vi "Main.vi"() -> ()   [LabVIEW 2011]
uses:
  typedefs/fiber_parameters_cluster.ctl
  fpga/typedefs/ramp_type_enum.ctl
  typedefs/spiral_parameters_cluster.ctl
  typedefs/run_parameters_cluster.ctl
  typedefs/run_mode_enum.ctl
  typedefs/acquisition_parameters_cluster.ctl
  typedefs/image_size_I32.ctl
  typedefs/scan_infos.ctl
  typedefs/smooth_coeffs_cluster.ctl
  typedefs/storage_parameters_cluster.ctl
  typedefs/mapping_corrections_cluster.ctl
  typedefs/pockels_corrections_cluster.ctl
  typedefs/fiber_parameters_pixelmapper_autoupdate_cluster.ctl
  typedefs/main_state_cluster.ctl
  typedefs/main_state_enum.ctl
  typedefs/control_process_state_cluster.ctl
  typedefs/control_process_state_enum.ctl
  typedefs/state_insert_position_enum.ctl
  <vilib>/Utility/error.llb/DialogType.ctl
  typedefs/all_scan_parameters_cluster.ctl
  <vilib>/DAQmx/write.llb/DAQmx Write (Digital Bool 1Line 1Point).vi
  globals/global_process_names.vi
  globals/global_exit.vi
  <vilib>/DAQmx/create/channels.llb/DAQmx Create Channel (DO-Digital Output).vi
  <vilib>/DAQmx/miscellaneous.llb/DAQmx Fill In Error Info.vi
  Fiberscope_library.lvlib
panel:
  out "Loaded process names":string[](array[string])
  in  "PMT":bool
  out "Version_string":string
  out "Loading":i32(slide) scale=0.0..6.0
  out "CPU":sgl(slide) scale=0.0..100.0
  in  "Comment":string
  in  "Save":bool
  in  "Start single":bool
  in  "Shutter":bool
  in  "Parameters":T1(tab)
  in  "Fiber parameters":T2={"Frequency"=2039.0, "Amplitude X"=0.3, "Amplitude Y"=0.3, "Initial Amplitude X"=0.0, "Initial Amplitude Y"=0.0, "Phase"=0.0, "Ramp type"=enum."Linear"} {"Phase" min=-90.0 max=90.0 step=5.0; "Initial Amplitude Y" min=0.0 max=1.0 step=0.1; "Initial Amplitude X" min=0.0 max=1.0 step=0.1; "Amplitude Y" min=0.0 max=4.0 step=0.1; "Amplitude X" min=0.0 max=4.0 step=0.1; "Frequency" min=100.0 max=6000.0 step=1.0}
  in  "Spiral parameters":T4={"Imaging periods"=100.0, "Settling periods"=50.0, "Resting periods"=100.0} {"Resting periods" min=10.0 max=1000.0 step=1.0; "Settling periods" min=1.0 max=1000.0 step=1.0; "Imaging periods" min=1.0 max=1000.0 step=1.0}
  in  "Run parameters":T5={"Run mode"=enum."Continuous", "Averages per frame"=1, "No. of frames"=1} {"No. of frames" min=1 max=1000 step=1; "Averages per frame" min=1 max=32}
  in  "Acquisition parameters":T7={"Cycles per pixel"=391, "Image size"=128, "Bidirectional acquisition"=FALSE} {"Image size" items=["128x128 px"=128, "256x256 px"=256, "512x512 px"=512]; "Cycles per pixel" min=100 max=90000 step=1}
  out "Scan infos":T9 {"Scan vs. Non-scan" scale=0.0..1.0}
  in  "Pockels corrections":T10 {"Delay pixels" min=0 max=10000 step=1}
  in  "Smoothing coefficients":T11 {"Coeff 1" min=0.0 max=1.0 step=0.05; "Coeff 2" min=0.0 max=1.0 step=0.05}
  in  "Fiber parameters pixelmapper":T2={"Frequency"=2039.0, "Amplitude X"=0.3, "Amplitude Y"=0.3, "Initial Amplitude X"=0.0, "Initial Amplitude Y"=0.0, "Phase"=0.0, "Ramp type"=enum."Linear"} {"Phase" min=-90.0 max=90.0 step=5.0; "Initial Amplitude Y" min=0.0 max=1.0 step=0.1; "Initial Amplitude X" min=0.0 max=1.0 step=0.1; "Amplitude Y" min=0.0 max=4.0 step=0.1; "Amplitude X" min=0.0 max=4.0 step=0.1; "Frequency" min=100.0 max=6000.0 step=1.0}
  in  "Mapping corrections":T12 {"Phase increase" min=-1.0 max=1.0 step=0.01}
  in  "Autoupdate":T13
  in  "Storage parameters":T14
  in  "PMT digital line":tag="PXI-6229/port0/line1"
  in  "Shutter digital line":tag="PXI-6229/port0/line0"
  in  "Start cont":bool
  in  "Quit":bool
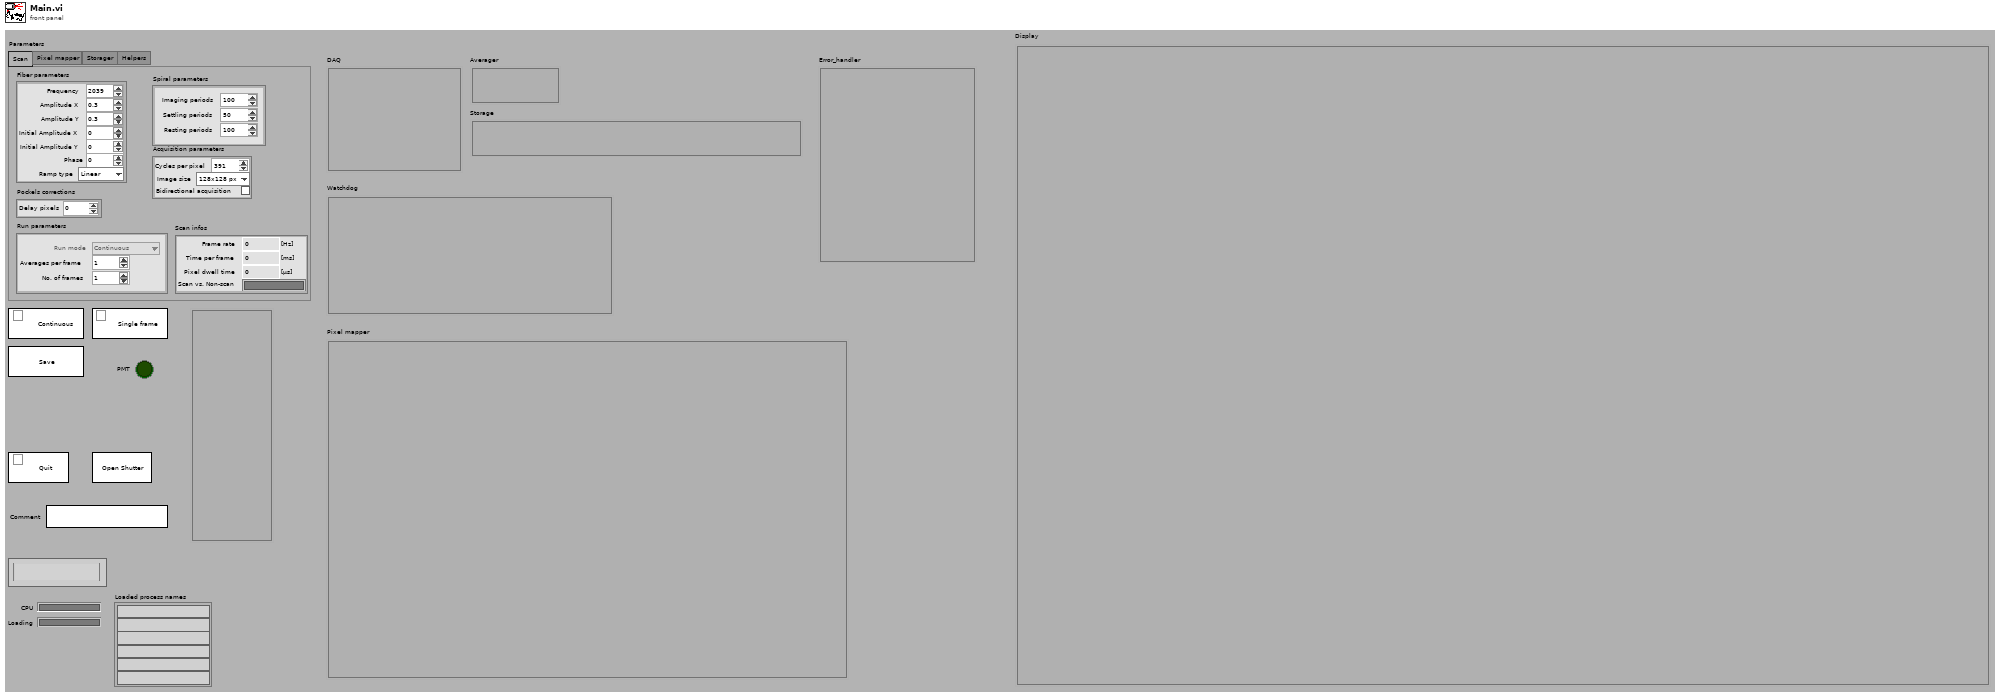
[diagram p1: front panel]
types:
  T1 = enum32{"Scan", "Pixel mapper", "Storager", "Helpers"}
  T2 = typedef "Fiberscope_library.lvlib/fiber_parameters_cluster.ctl" = cluster{"Frequency":dbl, "Amplitude X":dbl, "Amplitude Y":dbl, "Initial Amplitude X":dbl, "Initial Amplitude Y":dbl, "Phase":dbl, "Ramp type":T3}
  T3 = typedef "ramp_type_enum.ctl" = enum8{"Linear", "Sine"}
  T4 = typedef "Fiberscope_library.lvlib/spiral_parameters_cluster.ctl" = cluster{"Imaging periods":dbl, "Settling periods":dbl, "Resting periods":dbl}
  T5 = typedef "Fiberscope_library.lvlib/run_parameters_cluster.ctl" = cluster{"Run mode":T6, "Averages per frame":u8, "No. of frames":u32}
  T6 = typedef "Fiberscope_library.lvlib/run_mode_enum.ctl" = enum16{"Continuous", "Single frame", "No. of frames"}
  T7 = typedef "Fiberscope_library.lvlib/acquisition_parameters_cluster.ctl" = cluster{"Cycles per pixel":u32, "Image size":T8, "Bidirectional acquisition":bool}
  T8 = typedef "Fiberscope_library.lvlib/image_size_I32.ctl" = i32
  T9 = typedef "Fiberscope_library.lvlib/scan_infos.ctl" = cluster{"Frame rate":dbl, "Pixel dwell time":dbl, "Scan vs. Non-scan":dbl, "Time per frame":dbl}
  T10 = typedef "Fiberscope_library.lvlib/pockels_corrections_cluster.ctl" = cluster{"Delay pixels":i32}
  T11 = typedef "Fiberscope_library.lvlib/smooth_coeffs_cluster.ctl" = cluster{"Coeff 1":dbl, "Coeff 2":dbl}
  T12 = typedef "Fiberscope_library.lvlib/mapping_corrections_cluster.ctl" = cluster{"Phase increase":dbl, "Amplitude correction":dbl}
  T13 = typedef "Fiberscope_library.lvlib/fiber_parameters_pixelmapper_autoupdate_cluster.ctl" = cluster{"Frequency":bool, "Amplitude X":bool, "Amplitude Y":bool, "Initial Amplitude X":bool, "Initial Amplitude Y":bool, "Phase":bool, "Ramp type":bool}
  T14 = typedef "Fiberscope_library.lvlib/storage_parameters_cluster.ctl" = cluster{"Autosave":bool, "Path":path}
  T15 = typedef "Fiberscope_library.lvlib/main_state_cluster.ctl" = cluster{"Main_state_enum":T16, "State_data_variant":variant}
  T16 = typedef "Fiberscope_library.lvlib/main_state_enum.ctl" = enum16{"Init", "Error", "Quit", "Run", "Stop", "Change_parameters", "Timeout", "Shutter", "Save", "Wait_for_finished", "Change_storage", "Change_pixelmap", "Change_averages", "Run_finished", "Change_runmode", "PMT"}
  T17 = cluster{"Quit":refnum<vi>, "Start cont":refnum<vi>, "Parameters":refnum<vi>, "Fiber parameters":refnum<vi>, "Spiral parameters":refnum<vi>, "Run parameters":refnum<vi>, "Acquisition parameters":refnum<vi>, "Fiber parameters pixelmapper":refnum<vi>, "Shutter":refnum<vi>, "Save":refnum<vi>, "Comment":refnum<vi>, "Start single":refnum<vi>, "Storage parameters":refnum<vi>, "PMT":refnum<vi>}
  T18 = typedef "Fiberscope_library.lvlib/all_scan_parameters_cluster.ctl" = cluster{"Fiber parameters":T2, "Spiral parameters":T4, "Run parameters":T5, "Acquisition parameters":T7, "Fiber parameters pixel_mapper":T2, "Smooth_coeffs_cluster":T11, "Storage parameters":T14, "Mapping corrections":T12, "Pockels corrections":T10}
  T19 = cluster{"Mapping corrections":T12, "Smoothing coefficients":T11, "Fiber parameters pixelmapper":T2}
  T20 = typedef "Fiberscope_library.lvlib/control_process_state_cluster.ctl" = cluster{"Control_process_state_enum":T21, "variant":variant}
  T21 = typedef "Fiberscope_library.lvlib/control_process_state_enum.ctl" = enum16{"Init", "Quit", "Start", "Stop", "Change_parameters", "Running", "Finish", "Custom"}
  T22 = typedef "Fiberscope_library.lvlib/state_insert_position_enum.ctl" = enum16{"Insert_back", "Insert_front"}
  T23 = cluster{"error in (no error)":errorcluster, string}
  T24 = enum8{"Enabled", "Disabled", "Disabled and Grayed Out"}
  T25 = typedef "DialogType.ctl" = u16
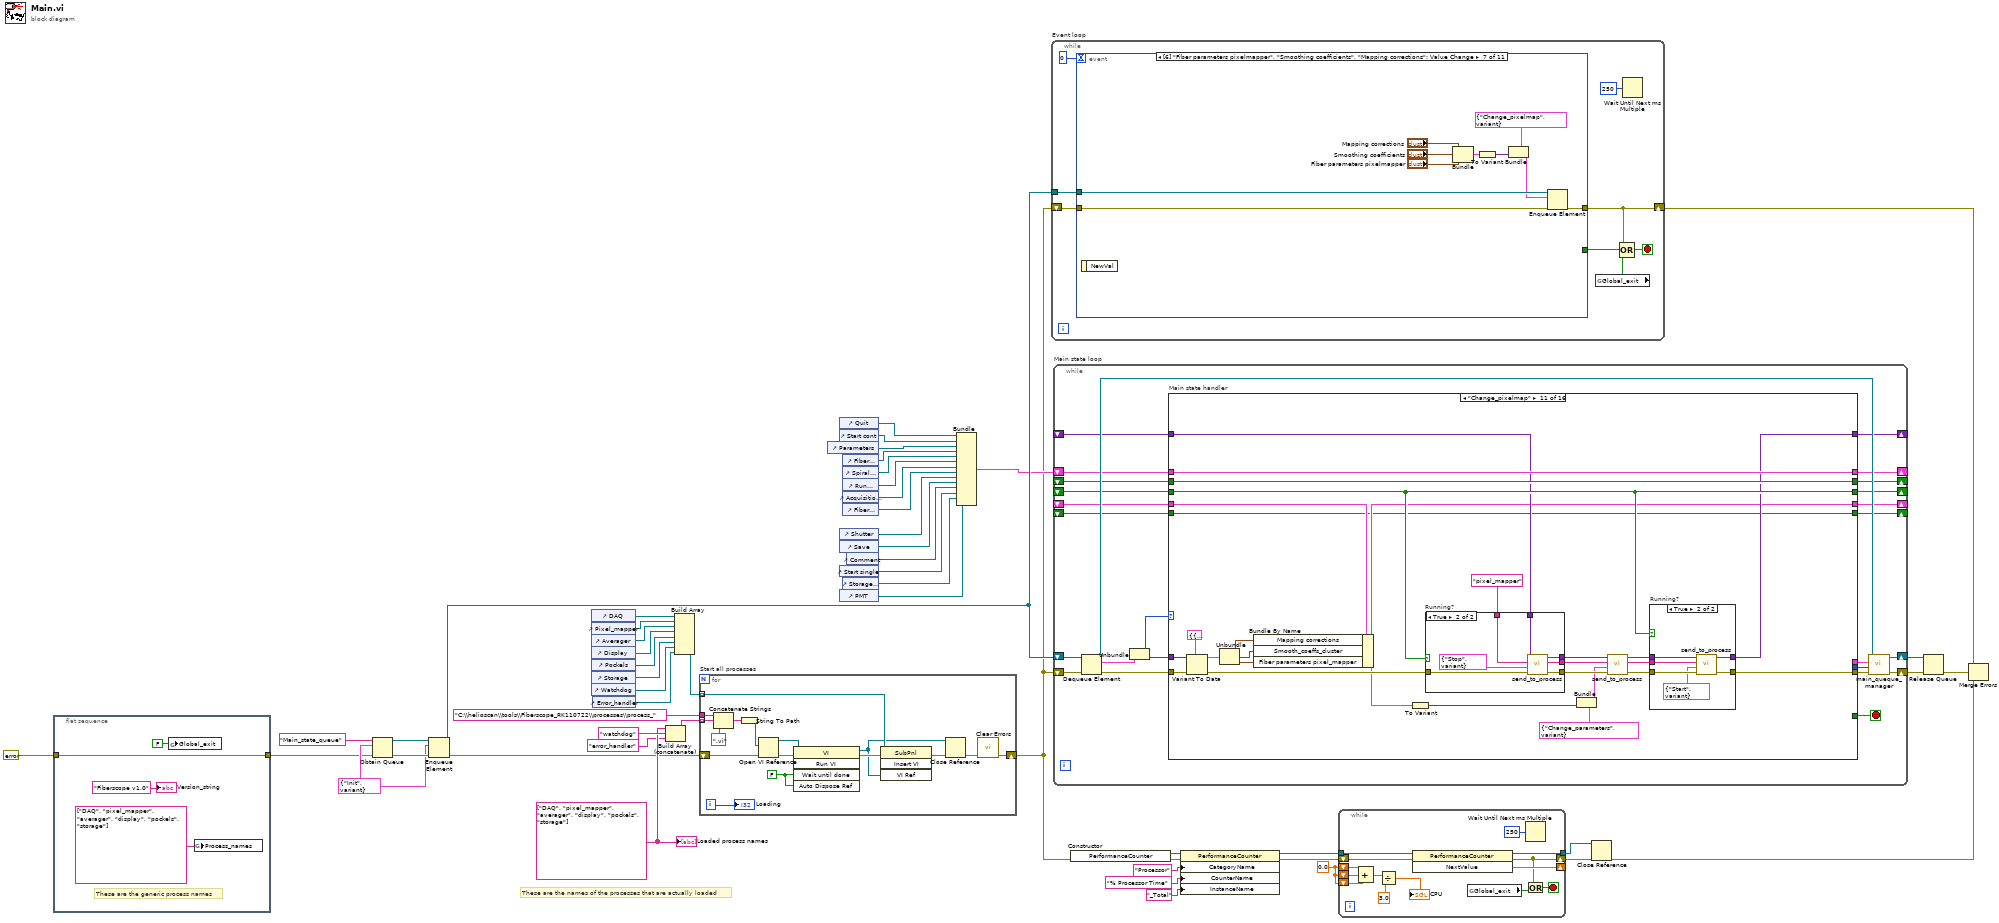
[diagram p0: block diagram]
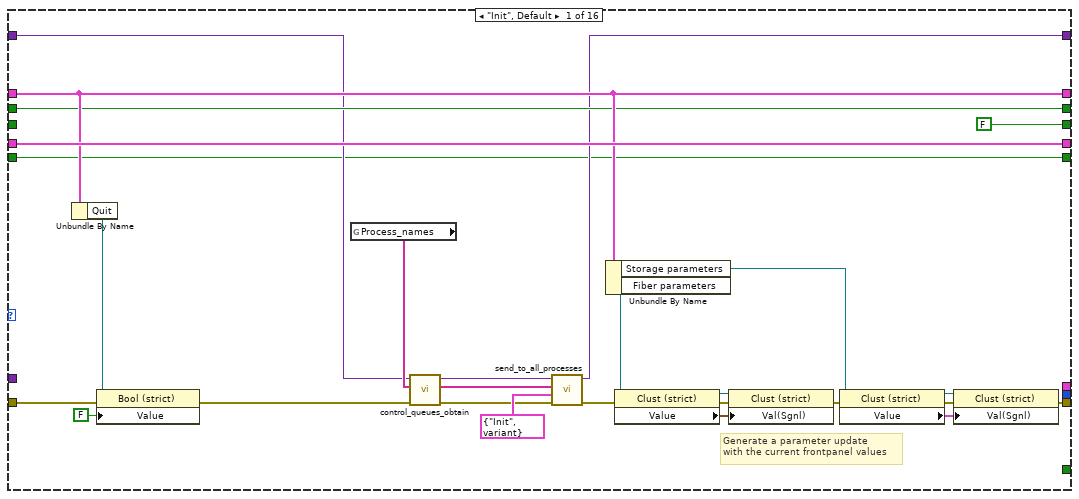
[diagram p2: hidden frame]
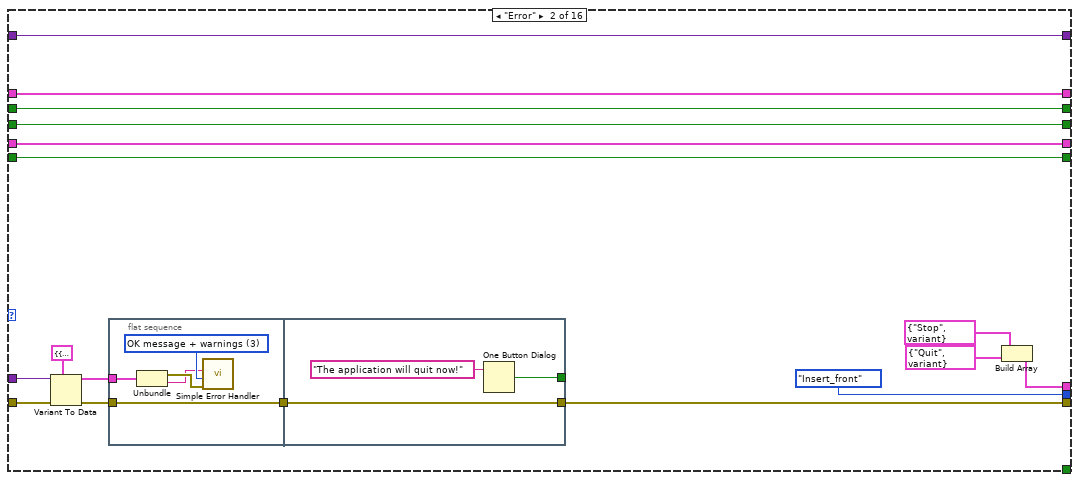
[diagram p3: hidden frame]
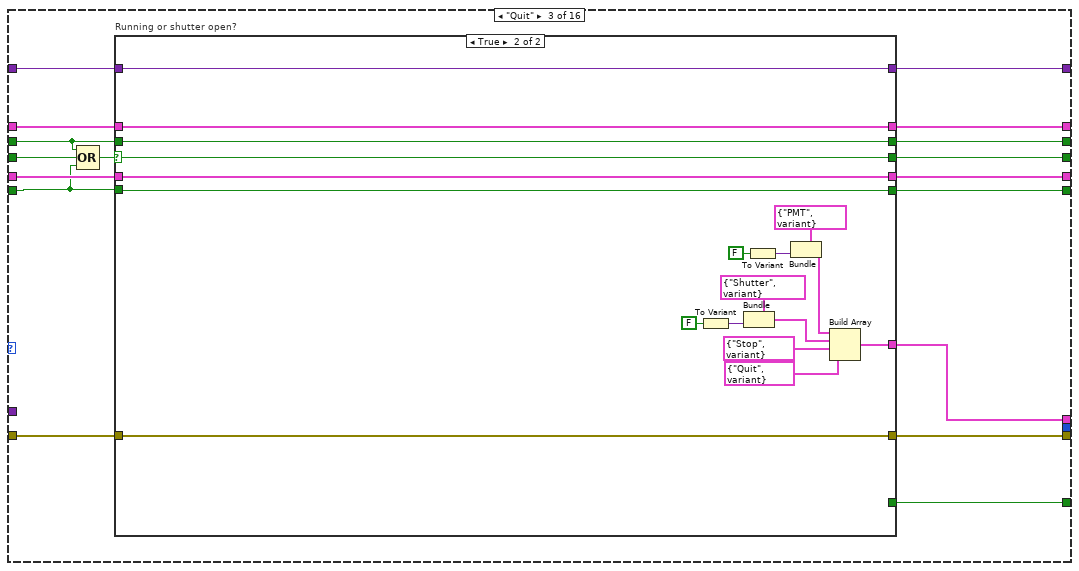
[diagram p4: hidden frame]
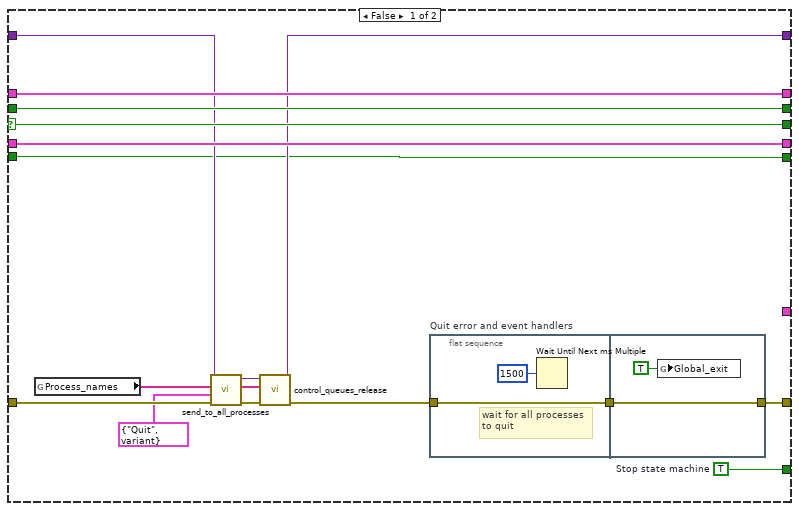
[diagram p5: hidden frame]
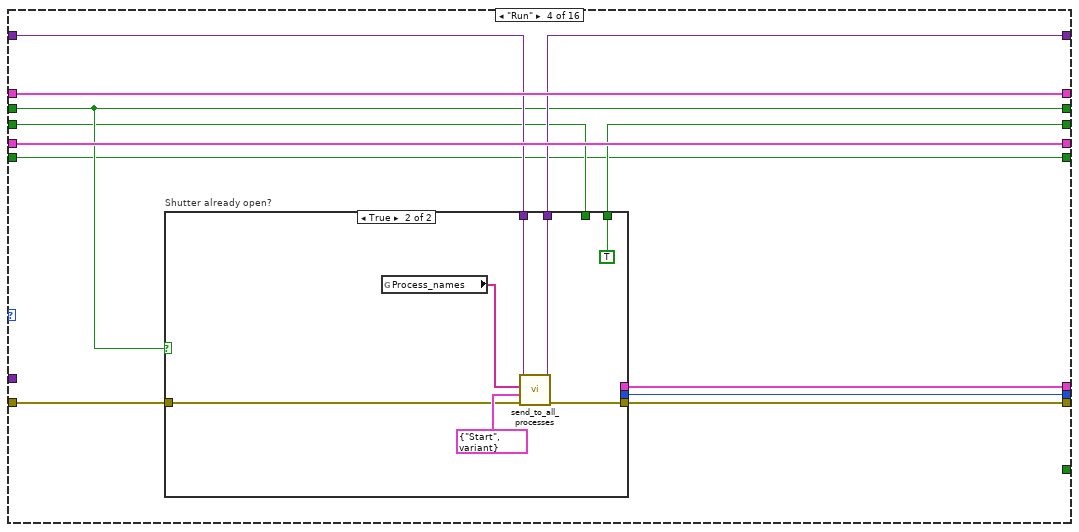
[diagram p6: hidden frame]
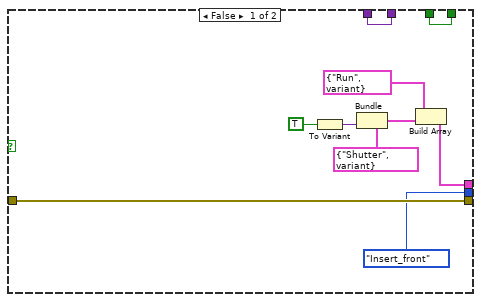
[diagram p7: hidden frame]
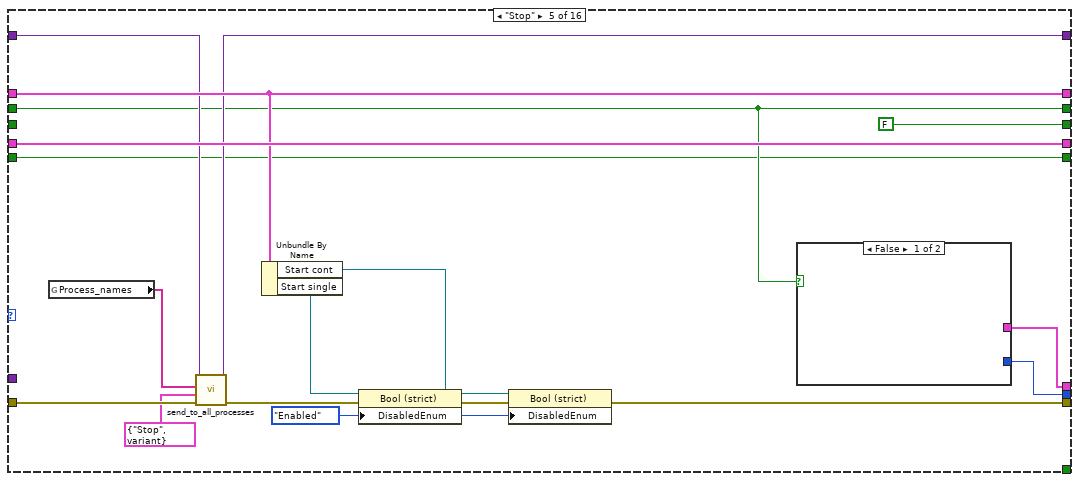
[diagram p8: hidden frame]
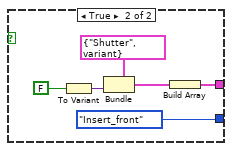
[diagram p9: hidden frame]
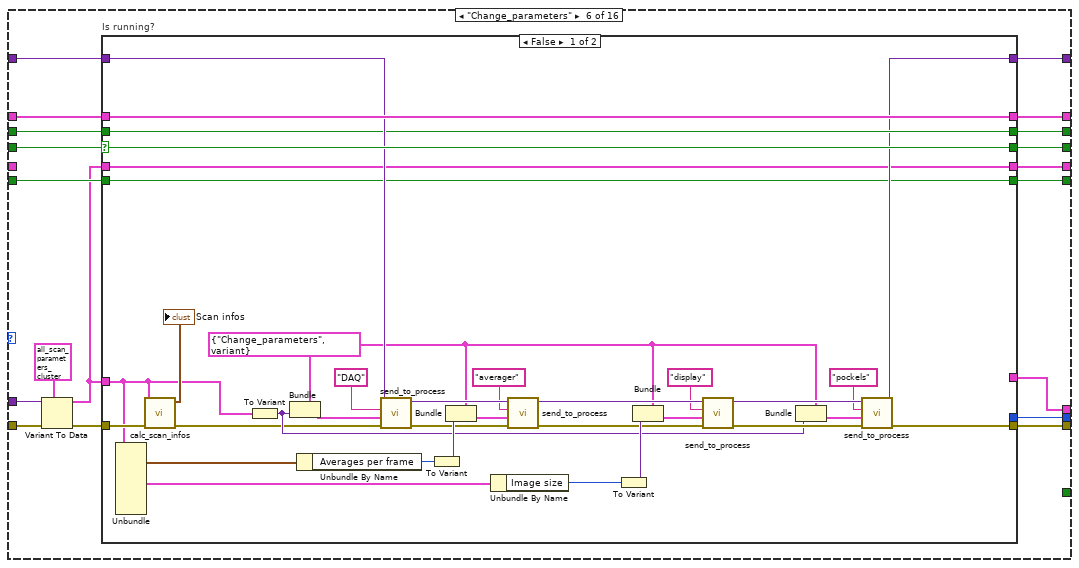
[diagram p10: hidden frame]
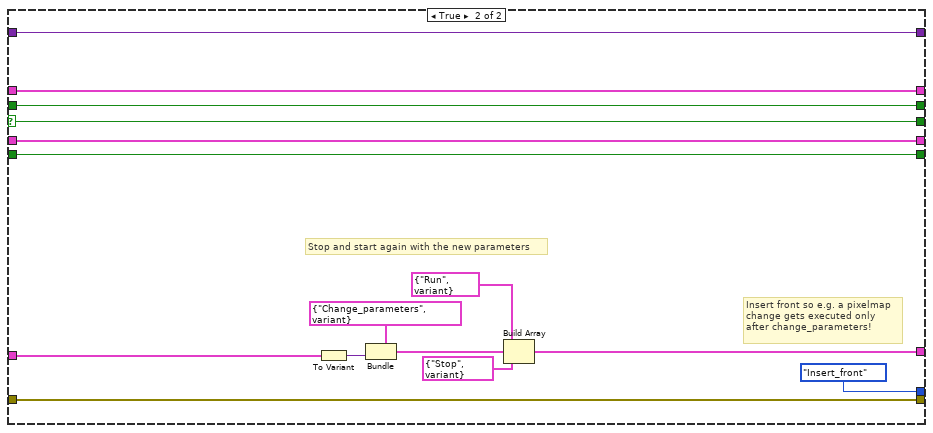
[diagram p11: hidden frame]
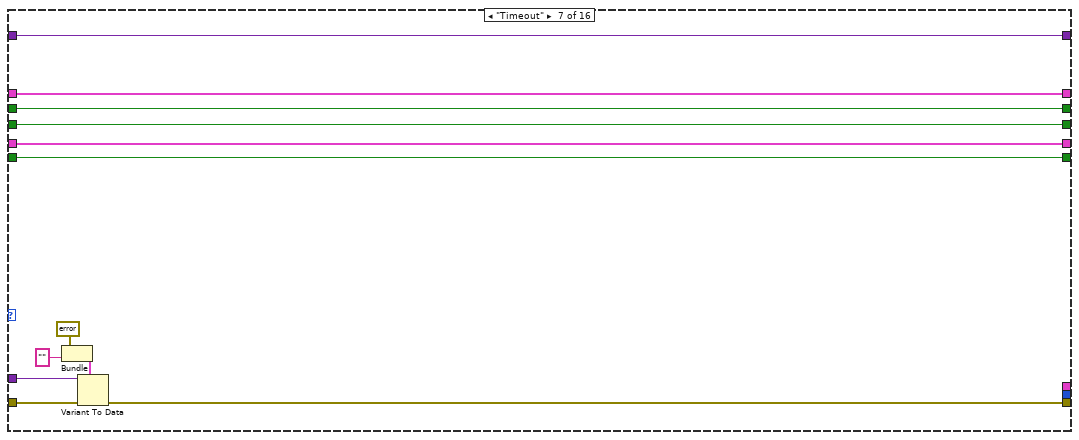
[diagram p12: hidden frame]
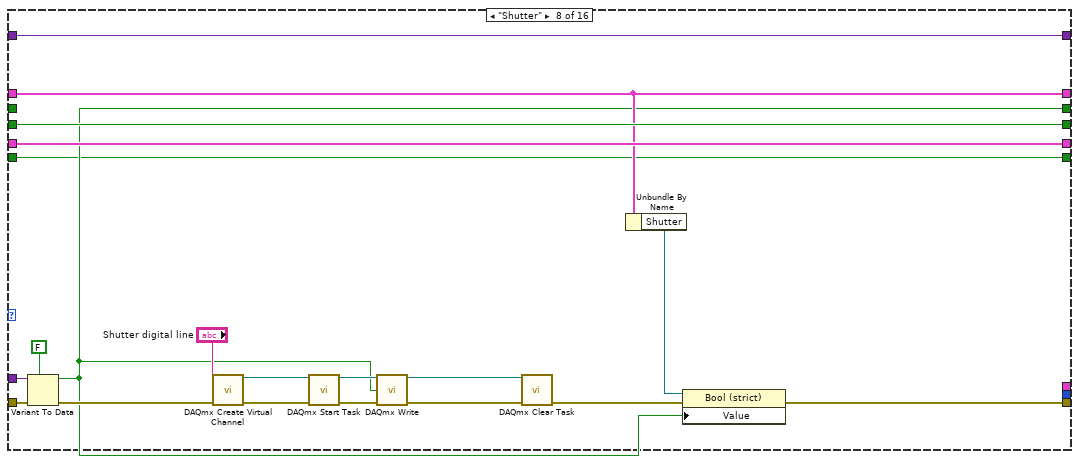
[diagram p13: hidden frame]
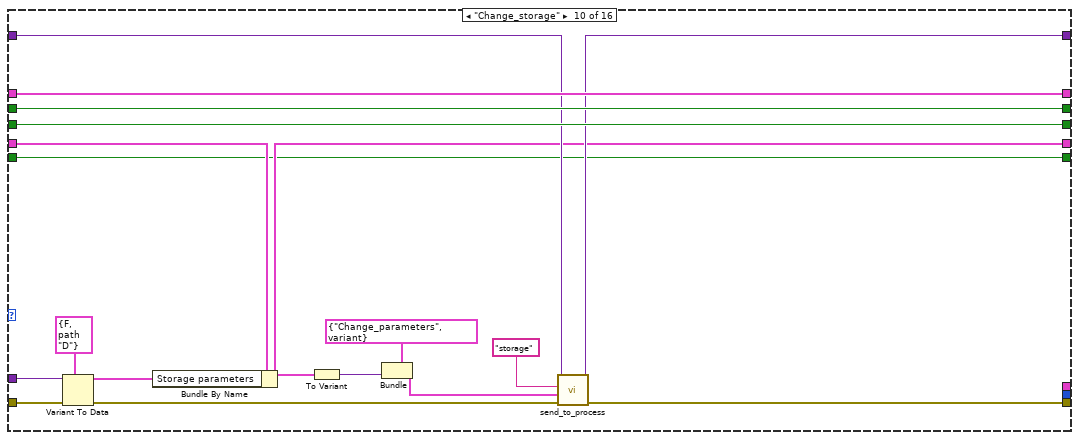
[diagram p15: hidden frame]
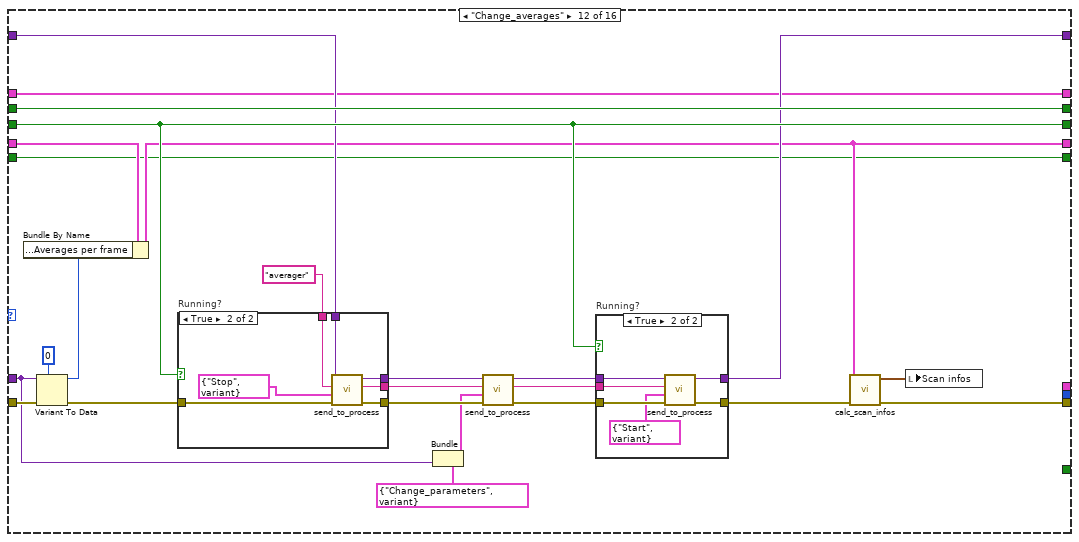
[diagram p18: hidden frame]
diagram:
  w10 = string[] ["DAQ", "pixel_mapper", "averager", "display", "pockels", "storage"]
  w22 = sgl 0.0 ("NextValue")
  w49 = T15 {"Main_state_enum"=enum."Init", "State_data_variant"=variant} ("Main_state_cluster")
  # "These are the names of the processes that are actually loaded"
  n1 = flat-sequence {
    tunnel: [w56] -> w37
    tunnel: errorcluster {"status"=FALSE, "code"=0, "source"=""} ("error in (no error)") -> [w56]
    frame #0 {
      # "These are the generic process names"
      n2 = global write "global_exit.vi" "Global_exit"(FALSE ("Global_exit")) -> ()
      n3 = global write "global_process_names.vi" "Process_names"(string[] ["DAQ", "pixel_mapper", "averager", "display", "pockels", "storage"]) -> ()
      "Version_string" <- "Fiberscope v1.0" ("Version_string")
    }
  }
  n4 = Obtain Queue(name (unnamed)="Main_state_queue", element data type=w49, error in (no error)=w37) -> (queue out=w51:refnum<queue>, error out=w52:errorcluster)  [unwired: 2 in, 1 out]
  n5 = Enqueue Element(queue=w51, element=w49, error in (no error)=w52) -> (queue out=w50:refnum<queue>, error out=w8:errorcluster)  [unwired: 1 in, 1 out]
  n6 = control-ref of="DAQ"() -> (w19:refnum<vi>)
  n7 = control-ref of="Pixel_mapper"() -> (w18:refnum<vi>)
  n8 = control-ref of="Averager"() -> (w17:refnum<vi>)
  n9 = control-ref of="Display"() -> (w16:refnum<vi>)
  n10 = control-ref of="Pockels"() -> (w14:refnum<vi>)
  n11 = control-ref of="Storage"() -> (w13:refnum<vi>)
  n12 = control-ref of="Watchdog"() -> (w12:refnum<vi>)
  n13 = control-ref of="Error_handler"() -> (w4:refnum<vi>)
  n14 = Build Array (concatenate)(w10, "watchdog", "error_handler" ("element")) -> (w9:string[])
  n15 = Build Array(w19, w18, w17, w16, w14, w13, w12, w4) -> (w15:refnum<vi>[])
  n16 = for "Start all processes" {
    tunnel: w9 -> [w71] mode=indexing
    tunnel: w15 -> [w73] mode=indexing
    tunnel: "C:\\helioscan\\tools\\Fiberscope_RK110722\\processes\\process_" -> [w72]
    shift-right: [w66] -> w6
    shift-left: w8 -> [w67]
    i -> [w58]
    w59 = FALSE
    n17 = Concatenate Strings(w72, w71, ".vi") -> (w69:string)
    n18 = String To Path(string=w69) -> (path=w68:path)
    n19 = Open VI Reference(vi path=w68, error in (no error)=w67) -> (vi reference=w61:refnum<vi>, error out=w63:errorcluster)  [unwired: 4 in]
    n20 = invoke class="VI" method="Run VI"(reference=w61, error in=w63, "Wait until done"=w59, "Auto Dispose Ref"=w59) -> (reference out=w60:refnum<vi>, error out=w62:errorcluster)  [unwired: 1 in, 3 out]
    n21 = invoke class="SubPnl" method="Insert VI"(reference=w73, error in=w62, "VI Ref"=w60) -> (error out=w65:errorcluster)  [unwired: 1 in, 3 out]
    n22 = Close Reference(reference=w60, error in (no error)=w65) -> (error out=w64:errorcluster)
    n23 = call <vilib>:"Clear Errors.vi"("error in (no error)"=w64) -> ("error out"=w66:errorcluster)  [unwired: 6 in]
    "Loading" <- w58
  }
  n24 = control-ref of="Parameters"() -> (w46:refnum<vi>)
  n25 = control-ref of="Quit"() -> (w48:refnum<vi>)
  n26 = control-ref of="Start cont"() -> (w47:refnum<vi>)
  n27 = control-ref of="Shutter"() -> (w34:refnum<vi>)
  n28 = control-ref of="Save"() -> (w33:refnum<vi>)
  n29 = control-ref of="Start single"() -> (w30:refnum<vi>)
  n30 = control-ref of="PMT"() -> (w1:refnum<vi>)
  n31 = control-ref of="Fiber parameters"() -> (w45:refnum<vi>)
  n32 = control-ref of="Spiral parameters"() -> (w44:refnum<vi>)
  n33 = control-ref of="Run parameters"() -> (w43:refnum<vi>)
  n34 = control-ref of="Acquisition parameters"() -> (w31:refnum<vi>)
  n35 = control-ref of="Fiber parameters pixelmapper"() -> (w35:refnum<vi>)
  n36 = control-ref of="Storage parameters"() -> (w3:refnum<vi>)
  n37 = control-ref of="Comment"() -> (w32:refnum<vi>)
  n38 = Bundle("Quit"=w48, "Start cont"=w47, "Parameters"=w46, "Fiber parameters"=w45, "Spiral parameters"=w44, "Run parameters"=w43, "Acquisition parameters"=w31, "Fiber parameters pixelmapper"=w35, "Shutter"=w34, "Save"=w33, "Comment"=w32, "Start single"=w30, "Storage parameters"=w3, "PMT"=w1) -> (w42:T17)  [unwired: 1 in]
  n39 = while "Event loop" {
    tunnel: w50 -> [w81]
    shift-right: [w74] -> w38
    shift-left: w6 -> [w80]
    stop <- w79 stop-if-true
    n40 = event shown="[6] \"Fiber parameters pixelmapper\", \"Smoothing coefficients\", \"Mapping corrections\": Value Change" {
      selector: _ -> [_ _ _ _ _ _ _ _ _ _ _]
      dyn-events: _ -> [_ _ _ _ _ _ _ _ _ _ _]
      timeout: 0 -> [_ _ _ _ _ _ _ _ _ _ _]
      tunnel: w81 -> [_ w84 w89 w113 w140 w145 w158 w161 w176 _ w184]
      tunnel: w80 -> [w82 w86 w90 w115 w125 w149 w150 w163 w178 w179 w186]
      tunnel: [w82 w85 w88 w114 w130 w146 w159 w162 w177 w179 w185] -> w74
      tunnel: [_ TRUE ("Quit") _ _ _ _ _ _ _ _ _] -> w78
      event Timeout {
        n41 = event-data() -> ()  [unwired: 1 in, 2 out]
      }
      event "Quit": Value Change {
        n42 = event-data() -> ()  [unwired: 1 in, 5 out]
        n43 = Enqueue Element(queue=w84, element=T15 {"Main_state_enum"=enum."Quit", "State_data_variant"=variant}, error in (no error)=w86) -> (error out=w85:errorcluster)  [unwired: 1 in, 2 out]
      }
      event "Start cont", "Start single": Value Change {
        n44 = event-data() -> ()  [unwired: 1 in, 5 out]
        n45 = Or(x="Start single", y="Start cont") -> (x .or. y?=w92:bool)
        n46 = Select(t=run_mode_enum."No. of frames" ("Run parameters.Run mode"), s="Start single", f=run_mode_enum."Continuous" ("Run parameters.Run mode")) -> (s? t:f=w91:T6)
        n47 = case "Start or stop?" shown="True" w92 {
          tunnel: w91 -> [_ w108]
          tunnel: w90 -> [w100 w107]
          tunnel: w89 -> [w98 w106]
          tunnel: [w99 w103] -> w88
          frame False {
            n48 = Enqueue Element(queue=w98, element=T15 {"Main_state_enum"=enum."Stop", "State_data_variant"=variant}, error in (no error)=w100) -> (error out=w99:errorcluster)  [unwired: 1 in, 2 out]
          }
          frame True {
            n49 = To Variant(anything=w108) -> (Variant=w109:variant)
            n50 = Bundle(cluster=T15 {"Main_state_enum"=enum."Change_runmode", "State_data_variant"=variant} ("element"), "State_data_variant"=w109) -> (w105:T15)  [unwired: 1 in]
            n51 = Enqueue Element(queue=w106, element=w105, error in (no error)=w107) -> (queue out=w102:refnum<queue>, error out=w104:errorcluster)  [unwired: 1 in, 1 out]
            n52 = Enqueue Element(queue=w102, element=T15 {"Main_state_enum"=enum."Run", "State_data_variant"=variant}, error in (no error)=w104) -> (error out=w103:errorcluster)  [unwired: 1 in, 2 out]
          }
        }
      }
      event Value Change {
        n53 = event-data() -> ()  [unwired: 1 in, 1 out]
        n54 = To Variant(anything="Storage parameters") -> (Variant=w116:variant)
        n55 = Bundle(cluster=T15 {"Main_state_enum"=enum."Change_storage", "State_data_variant"=variant} ("element"), "State_data_variant"=w116) -> (w112:T15)  [unwired: 1 in]
        n56 = Enqueue Element(queue=w113, element=w112, error in (no error)=w115) -> (error out=w114:errorcluster)  [unwired: 1 in, 2 out]
      }
      event Value Change {
        n57 = event-data() -> ()  [unwired: 1 in, 1 out]
        n58 = property on="Fiber prms pixelmapper" class="Clust (strict)"(error in=w125) -> (error out=w123:errorcluster, "Value"=w120:T2)  [unwired: 1 in, 1 out]
        n59 = call "autoupdate_fiber_parameters_pixelmapper.vi"("error in"=w123, "Autoupdate"="Autoupdate", "Fiber parameters"="Fiber parameters", "Fiber parameters pixelmapper in"=w120) -> ("error out"=w122:errorcluster, "Fiber parameters pixelmapper out"=w118:T2)  [unwired: 6 in]
        n60 = property on="Fiber prms pixelmapper" class="Clust (strict)"(error in=w122, "Val(Sgnl)"=w118) -> (error out=w124:errorcluster)  [unwired: 1 in, 1 out]
        n61 = property on="Smoothing coefficients" class="Clust (strict)"(error in=w124) -> (error out=w129:errorcluster, "Value"=w131:T11)  [unwired: 1 in, 1 out]
        n62 = property on="Mapping corrections" class="Clust (strict)"(error in=w129) -> (error out=w128:errorcluster, "Value"=w127:T12)  [unwired: 1 in, 1 out]
        n63 = Bundle(cluster=T18 {"Fiber parameters"={"Frequency"=100.0, "Amplitude X"=0.0, "Amplitude Y"=0.0, "Initial Amplitude X"=0.0, "Initial Amplitude Y"=0.0, "Phase"=0.0, "Ramp type"=enum."Linear"}, "Spiral parameters"={"Imaging periods"=1.0, "Settling periods"=1.0, "Resting periods"=1.0}, "Run parameters"={"Run mode"=enum."Continuous", "Averages per frame"=0, "No. of frames"=0}, "Acquisition parameters"={"Cycles per pixel"=0, "Image size"=1, "Bidirectional acquisition"=FALSE}, "Fiber parameters pixel_mapper"={"Frequency"=0.0, "Amplitude X"=0.0, "Amplitude Y"=0.0, "Initial Amplitude X"=0.0, "Initial Amplitude Y"=0.0, "Phase"=0.0, "Ramp type"=enum."Linear"}, "Smooth_coeffs_cluster"={"Coeff 1"=0.0, "Coeff 2"=0.0}, "Storage parameters"={"Autosave"=FALSE, "Path"=path ""}, "Mapping corrections"={"Phase increase"=0.0, "Amplitude correction"=0.0}, "Pockels corrections"={"Delay pixels"=0}} ("All scan parameters"), "Fiber parameters"="Fiber parameters", "Spiral parameters"="Spiral parameters", "Run parameters"="Run parameters", "Acquisition parameters"="Acquisition parameters", "Fiber parameters pixel_mapper"=w118, "Smooth_coeffs_cluster"=w131, "Mapping corrections"=w127, "Pockels corrections"="Pockels corrections") -> (w136:T18)  [unwired: 1 in]
        n64 = To Variant(anything=w136) -> (Variant=w138:variant)
        n65 = Bundle(cluster=T15 {"Main_state_enum"=enum."Change_parameters", "State_data_variant"=variant} ("element"), "State_data_variant"=w138) -> (w137:T15)  [unwired: 1 in]
        n66 = Enqueue Element(queue=w140, element=w137, error in (no error)=w128) -> (error out=w130:errorcluster)  [unwired: 1 in, 2 out]
      }
      event Value Change {
        n67 = event-data() -> ()  [unwired: 1 in, 1 out]
        n68 = property on="Run parameters" class="Clust (strict)"(error in=w149) -> (error out=w147:errorcluster, "Value"=w148:T5)  [unwired: 1 in, 1 out]
        n69 = Unbundle By Name(w148) -> ("Averages per frame"=w144:u8)
        n70 = To Variant(anything=w144) -> (Variant=w142:variant)
        n71 = Bundle(cluster=T15 {"Main_state_enum"=enum."Change_averages", "State_data_variant"=variant} ("element"), "State_data_variant"=w142) -> (w141:T15)  [unwired: 1 in]
        n72 = Enqueue Element(queue=w145, element=w141, error in (no error)=w147) -> (error out=w146:errorcluster)  [unwired: 1 in, 2 out]
      }
      event Value Change {
        n73 = event-data() -> ()  [unwired: 1 in, 1 out]
        n74 = Bundle("Mapping corrections"="Mapping corrections", "Smoothing coefficients"="Smoothing coefficients", "Fiber parameters pixelmapper"="Fiber parameters pixelmapper") -> (w153:T19)  [unwired: 1 in]
        n75 = To Variant(anything=w153) -> (Variant=w155:variant)
        n76 = Bundle(cluster=T15 {"Main_state_enum"=enum."Change_pixelmap", "State_data_variant"=variant} ("element"), "State_data_variant"=w155) -> (w156:T15)  [unwired: 1 in]
        n77 = Enqueue Element(queue=w158, element=w156, error in (no error)=w150) -> (error out=w159:errorcluster)  [unwired: 1 in, 2 out]
      }
      event "Save": Value Change {
        n78 = event-data() -> ()  [unwired: 1 in, 1 out]
        n79 = case "Save ON?" shown="True" "Save" {
          tunnel: w163 -> [w164 w171]
          tunnel: [w164 w170] -> w162
          tunnel: w161 -> [_ w169]
          frame False {
          }
          frame True {
            n80 = To Variant(anything="Comment") -> (Variant=w166:variant)
            n81 = Bundle(cluster=T15 {"Main_state_enum"=enum."Save", "State_data_variant"=variant} ("element"), "State_data_variant"=w166) -> (w167:T15)  [unwired: 1 in]
            n82 = Enqueue Element(queue=w169, element=w167, error in (no error)=w171) -> (error out=w170:errorcluster)  [unwired: 1 in, 2 out]
          }
        }
      }
      event "Shutter", "Shutter digital line": Value Change {
        n83 = event-data() -> ()  [unwired: 1 in, 5 out]
        n84 = To Variant(anything="Shutter") -> (Variant=w174:variant)
        n85 = Bundle(cluster=T15 {"Main_state_enum"=enum."Shutter", "State_data_variant"=variant} ("Main_state_cluster"), "State_data_variant"=w174) -> (w173:T15)  [unwired: 1 in]
        n86 = Enqueue Element(queue=w176, element=w173, error in (no error)=w178) -> (error out=w177:errorcluster)  [unwired: 1 in, 2 out]
      }
      event "Parameters": Value Change {
        # "Dummy case"
        n87 = event-data() -> ()  [unwired: 1 in, 5 out]
      }
      event "PMT": Value Change {
        n88 = event-data() -> ()  [unwired: 1 in, 5 out]
        n89 = To Variant(anything="PMT") -> (Variant=w182:variant)
        n90 = Bundle(cluster=T15 {"Main_state_enum"=enum."PMT", "State_data_variant"=variant} ("element"), "State_data_variant"=w182) -> (w180:T15)  [unwired: 1 in]
        n91 = Enqueue Element(queue=w184, element=w180, error in (no error)=w186) -> (error out=w185:errorcluster)  [unwired: 1 in, 2 out]
      }
    }
    n92 = global read "global_exit.vi" "Global_exit"() -> (w76:bool)
    n93 = Compound Arithmetic op=OR(w74, w78, w76) -> (w79:bool)
    n94 = Wait Until Next ms Multiple(millisecond multiple=u32 250) -> ()  [unwired: 1 out]
  }
  n95 = while "Main state loop" {
    shift-right: [w204] -> w41
    shift-left: w6 -> [w211]
    shift-right: [w199] -> _
    shift-left: _ -> [w198]
    shift-right: [w203] -> w40
    shift-left: w50 -> [w210]
    shift-right: [w197] -> _
    shift-left: w42 -> [w200]
    shift-right: [w193] -> _
    shift-left: _ -> [w194]
    shift-right: [w192] -> _
    shift-left: _ -> [w191]
    shift-right: [w190] -> _
    shift-left: _ -> [w189]
    shift-right: [w188] -> _
    shift-left: _ -> [w187]
    stop <- w196 stop-if-true
    n96 = Dequeue Element(queue=w210, error in (no error)=w211) -> (queue out=w202:refnum<queue>, element=w209:T15, error out=w208:errorcluster)  [unwired: 1 in, 1 out]
    n97 = Unbundle(w209) -> ("Main_state_enum"=w206:T16, "State_data_variant"=w207:variant)
    n98 = case "Main state handler" shown="\"Change_pixelmap\"" w206 {
      tunnel: w208 -> [w229 w254 w279 w327 w361 w389 w444 w469 w473 w486 w506 w562 w598 w612 w632 w651]
      tunnel: [w215 w245 w274 w326 w362 w383 w448 w454 w473 w491 w520 w543 w592 w609 w626 w638] -> w205
      tunnel: w207 -> [_ w253 _ _ _ w388 w443 w468 _ w484 w504 w559 w597 _ w631 w650]
      tunnel: [_ w251 w275 w322 w350 w385 _ _ _ _ _ _ _ w606 _ _] -> w201
      tunnel: w200 -> [w231 w249 w277 w328 w363 w382 w449 w456 w476 w495 w521 w542 w593 w614 w634 w640]
      tunnel: [FALSE w250 w278 w321 FALSE w386 w450 w470 w477 w494 w519 w556 w599 FALSE w635 w655] -> w199
      tunnel: w198 -> [_ w250 w268 w319 _ w387 w450 w470 w477 w494 w519 w556 w599 _ w635 w655]
      tunnel: [w231 w249 w276 w328 w363 w381 w449 w456 w476 w495 w521 w542 w593 w614 w634 w640] -> w197
      tunnel: [_ _ w273 _ _ _ _ _ _ _ _ _ _ _ _ _] -> w196
      tunnel: [_ state_insert_position_enum."Insert_front" ("State_insert_position_enum") _ w320 w349 w376 _ _ _ _ _ _ _ _ _ _] -> w195
      tunnel: [w225 w241 w271 w324 w359 w379 w442 w460 w474 w487 w507 w545 w582 w617 w624 w654] -> w193
      tunnel: w194 -> [w221 w241 w272 w325 w360 w380 w442 w460 w474 w489 w512 w550 w583 w617 w625 w654]
      tunnel: [w232 w240 w269 w329 w364 w378 w441 w459 w475 w479 w501 w541 w595 w616 w619 w653] -> w192
      tunnel: w191 -> [w232 w240 w270 w329 w364 _ w441 w459 w475 w481 w503 w557 w595 w616 w628 w653]
      tunnel: [w228 w239 w265 w323 w348 w374 w440 w452 w472 w493 w517 w555 w589 w615 w633 w652] -> w190
      tunnel: w189 -> [w228 w239 w266 w323 w348 w375 w440 _ w472 w493 w517 w555 w589 w615 w633 w652]
      tunnel: [w213 w238 w263 w318 w347 w372 w439 w451 w471 w478 w496 w539 w580 w600 w618 w636] -> w188
      tunnel: w187 -> [w213 w238 w264 w318 w347 w373 w439 w451 w471 w478 w496 w539 w580 w600 w618 _]
      frame "Init", Default {
        # "Generate a parameter update\nwith the current frontpanel values"
        n99 = Unbundle By Name(w231) -> ("Quit"=w230:refnum<vi>)
        n100 = property class="Bool (strict)"(reference=w230, error in=w229, "Value"=FALSE) -> (error out=w212:errorcluster)  [unwired: 1 out]
        n101 = global read "global_process_names.vi" "Process_names"() -> (w224:string[])
        n102 = call "control_queues_obtain.vi"("error in"=w212, "Process names in"=w224, "Process_communication in"=w221) -> ("error out"=w222:errorcluster, "Process_communication out"=w223:variant)  [unwired: 5 in]
        n103 = call "send_to_all_processes.vi"("error in (no error)"=w222, "Control_process_state_cluster in"=T20 {"Control_process_state_enum"=enum."Init", "variant"=variant}, "Process names"=w224, "Process_communication in"=w223) -> ("error out"=w227:errorcluster, "Process_communication out"=w225:variant)  [unwired: 6 in]
        n104 = Unbundle By Name(w231) -> ("Storage parameters"=w214:refnum<vi>, "Fiber parameters"=w234:refnum<vi>)
        n105 = property class="Clust (strict)"(reference=w234, error in=w227) -> (reference out=w233:refnum<vi>, error out=w235:errorcluster, "Value"=w236:T2)
        n106 = property class="Clust (strict)"(reference=w233, error in=w235, "Val(Sgnl)"=w236) -> (error out=w219:errorcluster)  [unwired: 1 out]
        n107 = property class="Clust (strict)"(reference=w214, error in=w219) -> (reference out=w216:refnum<vi>, error out=w218:errorcluster, "Value"=w217:T14)
        n108 = property class="Clust (strict)"(reference=w216, error in=w218, "Val(Sgnl)"=w217) -> (error out=w215:errorcluster)  [unwired: 1 out]
      }
      frame "Error" {
        n109 = Variant To Data(error in=w254, type=T23 {"error in (no error)"={"status"=FALSE, "code"=0, "source"=""}, ""}, Variant=w253) -> (data=w246:T23, error out=w248:errorcluster)
        n110 = flat-sequence {
          tunnel: w248 -> [w259]
          tunnel: [w259] -> w247
          tunnel: w246 -> [w257]
          tunnel: [w262] -> w245
          tunnel: [w260] -> _
          tunnel: w247 -> [w262]
          frame #0 {
            w258 = T25 3 items=["no dialog", "OK message", "continue or stop message", "OK message + warnings", "continue/stop + warnings"] ("type of dialog (OK msg:1)")
            n111 = Unbundle(w257) -> ("error in (no error)"=w256:errorcluster, w255:string)
            n112 = call <vilib>:"Simple Error Handler.vi"("error source (\" \")"=w255, "type of dialog (OK msg:1)"=w258, "error in (no error)"=w256) -> ()  [unwired: 2 in, 5 out]
          }
          frame #1 {
            n113 = One Button Dialog(message="The application will quit now!") -> (true=w260:bool)  [unwired: 1 in]
          }
        }
        n114 = Build Array(T15 {"Main_state_enum"=enum."Stop", "State_data_variant"=variant} ("element"), T15 {"Main_state_enum"=enum."Quit", "State_data_variant"=variant} ("Main_state_cluster")) -> (w251:T15[])
      }
      frame "Quit" {
        n115 = Compound Arithmetic op=OR(w266, w268, w264) -> (w267:bool)
        n116 = case "Running or shutter open?" shown="True" w267 {
          selector: w267 -> [w295 w316]
          tunnel: w279 -> [w287 w312]
          tunnel: [w293 w312] -> w274
          tunnel: [w295 w316] -> w278
          tunnel: [w294 w317] -> w276
          tunnel: w277 -> [w294 w317]
          tunnel: [_ w313] -> w275
          tunnel: [w292 _] -> w273
          tunnel: w272 -> [w285 w311]
          tunnel: [w282 w311] -> w271
          tunnel: w270 -> [w290 w310]
          tunnel: [w290 w310] -> w269
          tunnel: w266 -> [w289 w309]
          tunnel: [w289 w309] -> w265
          tunnel: w264 -> [w280 w300]
          tunnel: [w280 w300] -> w263
          frame False {
            w292 = TRUE  # Stop state machine
            n117 = global read "global_process_names.vi" "Process_names"() -> (w283:string[])
            n118 = call "send_to_all_processes.vi"("error in (no error)"=w287, "Control_process_state_cluster in"=T20 {"Control_process_state_enum"=enum."Quit", "variant"=variant}, "Process names"=w283, "Process_communication in"=w285) -> ("error out"=w288:errorcluster, "Process_communication out"=w284:variant)  [unwired: 6 in]
            n119 = call "control_queues_release.vi"("error in"=w288, "Process names in"=w283, "Process_communication in"=w284) -> ("error out"=w281:errorcluster, "Process_communication out"=w282:variant)  [unwired: 7 in]
            n120 = flat-sequence "Quit error and event handlers" {
              tunnel: w281 -> [w297]
              tunnel: [w297] -> w291
              tunnel: [w299] -> w293
              tunnel: w291 -> [w299]
              frame #0 {
                # "wait for all processes\nto quit"
                n121 = Wait Until Next ms Multiple(millisecond multiple=u32 1500) -> ()  [unwired: 1 out]
              }
              frame #1 {
                n122 = global write "global_exit.vi" "Global_exit"(TRUE ("Global_exit")) -> ()
              }
            }
          }
          frame True {
            n123 = To Variant(anything=FALSE) -> (Variant=w307:variant)
            n124 = Bundle(cluster=T15 {"Main_state_enum"=enum."Shutter", "State_data_variant"=variant} ("element"), "State_data_variant"=w307) -> (w305:T15)  [unwired: 1 in]
            n125 = To Variant(anything=FALSE) -> (Variant=w303:variant)
            n126 = Bundle(cluster=T15 {"Main_state_enum"=enum."PMT", "State_data_variant"=variant} ("element"), "State_data_variant"=w303) -> (w301:T15)  [unwired: 1 in]
            n127 = Build Array(w301, w305, T15 {"Main_state_enum"=enum."Stop", "State_data_variant"=variant} ("Main_state_cluster"), T15 {"Main_state_enum"=enum."Quit", "State_data_variant"=variant} ("Main_state_cluster")) -> (w313:T15[])
          }
        }
      }
      frame "Run" {
        n128 = case "Shutter already open?" shown="True" w323 {
          tunnel: w327 -> [w338 w340]
          tunnel: [w338 w346] -> w326
          tunnel: w325 -> [w339 w345]
          tunnel: [w339 w343] -> w324
          tunnel: [w337 _] -> w322
          tunnel: [w330 TRUE] -> w321
          tunnel: [state_insert_position_enum."Insert_front" ("State_insert_position_enum") _] -> w320
          tunnel: w319 -> [w330 _]
          frame False {
            n129 = To Variant(anything=TRUE) -> (Variant=w334:variant)
            n130 = Bundle(cluster=T15 {"Main_state_enum"=enum."Shutter", "State_data_variant"=variant} ("Main_state_cluster"), "State_data_variant"=w334) -> (w332:T15)  [unwired: 1 in]
            n131 = Build Array(T15 {"Main_state_enum"=enum."Run", "State_data_variant"=variant} ("Main_state_cluster"), w332) -> (w337:T15[])
          }
          frame True {
            n132 = global read "global_process_names.vi" "Process_names"() -> (w342:string[])
            n133 = call "send_to_all_processes.vi"("error in (no error)"=w340, "Control_process_state_cluster in"=T20 {"Control_process_state_enum"=enum."Start", "variant"=variant}, "Process names"=w342, "Process_communication in"=w345) -> ("error out"=w346:errorcluster, "Process_communication out"=w343:variant)  [unwired: 6 in]
          }
        }
      }
      frame "Stop" {
        w354 = T24."Enabled" ("Disabled")
        n134 = global read "global_process_names.vi" "Process_names"() -> (w351:string[])
        n135 = call "send_to_all_processes.vi"("error in (no error)"=w361, "Control_process_state_cluster in"=T20 {"Control_process_state_enum"=enum."Stop", "variant"=variant}, "Process names"=w351, "Process_communication in"=w360) -> ("error out"=w353:errorcluster, "Process_communication out"=w359:variant)  [unwired: 6 in]
        n136 = Unbundle By Name(w363) -> ("Start cont"=w355:refnum<vi>, "Start single"=w356:refnum<vi>)
        n137 = property class="Bool (strict)"(reference=w356, error in=w353, "DisabledEnum"=w354) -> (error out=w357:errorcluster)  [unwired: 1 out]
        n138 = property class="Bool (strict)"(reference=w355, error in=w357, "DisabledEnum"=w354) -> (error out=w362:errorcluster)  [unwired: 1 out]
        n139 = case shown="False" w348 {
          tunnel: [_ w366] -> w350
          tunnel: [_ state_insert_position_enum."Insert_front" ("State_insert_position_enum")] -> w349
          frame False {
          }
          frame True {
            n140 = To Variant(anything=FALSE) -> (Variant=w368:variant)
            n141 = Bundle(cluster=T15 {"Main_state_enum"=enum."Shutter", "State_data_variant"=variant} ("Main_state_cluster"), "State_data_variant"=w368) -> (w370:T15)  [unwired: 1 in]
            n142 = Build Array(w370) -> (w366:T15[])
          }
        }
      }
      frame "Change_parameters" {
        n143 = Variant To Data(error in=w389, type=T18 {"Fiber parameters"={"Frequency"=100.0, "Amplitude X"=0.0, "Amplitude Y"=0.0, "Initial Amplitude X"=0.0, "Initial Amplitude Y"=0.0, "Phase"=0.0, "Ramp type"=enum."Linear"}, "Spiral parameters"={"Imaging periods"=1.0, "Settling periods"=1.0, "Resting periods"=1.0}, "Run parameters"={"Run mode"=enum."Continuous", "Averages per frame"=0, "No. of frames"=0}, "Acquisition parameters"={"Cycles per pixel"=0, "Image size"=1, "Bidirectional acquisition"=FALSE}, "Fiber parameters pixel_mapper"={"Frequency"=0.0, "Amplitude X"=0.0, "Amplitude Y"=0.0, "Initial Amplitude X"=0.0, "Initial Amplitude Y"=0.0, "Phase"=0.0, "Ramp type"=enum."Linear"}, "Smooth_coeffs_cluster"={"Coeff 1"=0.0, "Coeff 2"=0.0}, "Storage parameters"={"Autosave"=FALSE, "Path"=path ""}, "Mapping corrections"={"Phase increase"=0.0, "Amplitude correction"=0.0}, "Pockels corrections"={"Delay pixels"=0}} ("All scan parameters"), Variant=w388) -> (data=w371:T18, error out=w384:errorcluster)
        n144 = case "Is running?" shown="False" w387 {
          selector: w387 -> [w423 w433]
          tunnel: w371 -> [w392 w437]
          tunnel: [w423 w433] -> w386
          tunnel: [_ w435] -> w385
          tunnel: w384 -> [w395 w432]
          tunnel: [w402 w432] -> w383
          tunnel: [w422 w431] -> w381
          tunnel: w382 -> [w422 w431]
          tunnel: w380 -> [w410 w430]
          tunnel: [w400 w430] -> w379
          tunnel: [w390 w424] -> w378
          tunnel: w371 -> [w390 w424]
          tunnel: [_ state_insert_position_enum."Insert_front" ("State_insert_position_enum")] -> w376
          tunnel: w375 -> [w404 w426]
          tunnel: [w404 w426] -> w374
          tunnel: [w391 w425] -> w372
          tunnel: w373 -> [w391 w425]
          frame False {
            w397 = T20 {"Control_process_state_enum"=enum."Change_parameters", "variant"=variant} ("Control_process_state_cluster")
            n145 = Unbundle(w392) -> ("Run parameters"=w420:T5, "Acquisition parameters"=w418:T7)  [unwired: 7 out]
            n146 = call "calc_scan_infos.vi"("error in"=w395, "All scan parameters"=w392) -> ("error out"=w394:errorcluster, "Scan infos"=→"Scan infos":T9)  [unwired: 8 in]
            n147 = To Variant(anything=w392) -> (Variant=w396:variant)
            n148 = Bundle(cluster=w397, "variant"=w396) -> (w415:T20)  [unwired: 1 in]
            n149 = Unbundle By Name(w420) -> ("Averages per frame"=w419:u8)
            n150 = call "send_to_process.vi"("error in"=w394, "Control_process_state_cluster in"=w415, "Process name"="DAQ", "Process_communication in"=w410) -> ("error out"=w413:errorcluster, "Process_communication out"=w408:variant)  [unwired: 6 in]
            n151 = To Variant(anything=w419) -> (Variant=w421:variant)
            n152 = Bundle(cluster=w397, "variant"=w421) -> (w414:T20)  [unwired: 1 in]
            n153 = Unbundle By Name(w418) -> ("Image size"=w416:T8)
            n154 = call "send_to_process.vi"("error in"=w413, "Control_process_state_cluster in"=w414, "Process name"="averager", "Process_communication in"=w408) -> ("error out"=w411:errorcluster, "Process_communication out"=w406:variant)  [unwired: 6 in]
            n155 = To Variant(anything=w416) -> (Variant=w417:variant)
            n156 = Bundle(cluster=w397, "variant"=w417) -> (w412:T20)  [unwired: 1 in]
            n157 = call "send_to_process.vi"("error in"=w411, "Control_process_state_cluster in"=w412, "Process name"="display", "Process_communication in"=w406) -> ("error out"=w403:errorcluster, "Process_communication out"=w401:variant)  [unwired: 6 in]
            n158 = Bundle(cluster=w397, "variant"=w396) -> (w398:T20)  [unwired: 1 in]
            n159 = call "send_to_process.vi"("error in"=w403, "Control_process_state_cluster in"=w398, "Process name"="pockels", "Process_communication in"=w401) -> ("error out"=w402:errorcluster, "Process_communication out"=w400:variant)  [unwired: 6 in]
          }
          frame True {
            # "Insert front so e.g. a pixelmap\nchange gets executed only\nafter change_parameters!"
            # "Stop and start again with the new parameters"
            n160 = To Variant(anything=w437) -> (Variant=w438:variant)
            n161 = Bundle(cluster=T15 {"Main_state_enum"=enum."Change_parameters", "State_data_variant"=variant} ("Main_state_cluster"), "State_data_variant"=w438) -> (w434:T15)  [unwired: 1 in]
            n162 = Build Array(T15 {"Main_state_enum"=enum."Run", "State_data_variant"=variant} ("Main_state_cluster"), w434, T15 {"Main_state_enum"=enum."Stop", "State_data_variant"=variant} ("Main_state_cluster")) -> (w435:T15[])
          }
        }
      }
      frame "Timeout" {
        n163 = Bundle("error out"=errorcluster {"status"=FALSE, "code"=0, "source"=""}, "") -> (w445:cluster{"error out":errorcluster, string})  [unwired: 1 in]
        n164 = Variant To Data(error in=w444, type=w445, Variant=w443) -> (error out=w448:errorcluster)  [unwired: 1 out]
      }
      frame "Shutter" {
        n165 = Variant To Data(error in=w469, type=FALSE ("Shutter"), Variant=w468) -> (data=w452:bool, error out=w461:errorcluster)
        n166 = call-poly <vilib>:"DAQmx Create Virtual Channel.vi"("lines"="Shutter digital line", "error in"=w461) -> ("task out"=w467:refnum<k21>, "error out"=w466:errorcluster)  [unwired: 12 in]
        n167 = call <vilib>:"DAQmx Start Task.vi"("task/channels in"=w467, "error in"=w466) -> ("task out"=w465:refnum<k21>, "error out"=w464:errorcluster)  [unwired: 12 in]
        n168 = call-poly <vilib>:"DAQmx Write.vi"("task/channels in"=w465, "data"=w452, "error in"=w464) -> ("task out"=w463:refnum<k21>, "error out"=w462:errorcluster)  [unwired: 10 in, 1 out]
        n169 = call <vilib>:"DAQmx Clear Task.vi"("task in"=w463, "error in"=w462) -> ("error out"=w455:errorcluster)  [unwired: 13 in]
        n170 = Unbundle By Name(w456) -> ("Shutter"=w453:refnum<vi>)
        n171 = property class="Bool (strict)"(reference=w453, error in=w455, "Value"=w452) -> (error out=w454:errorcluster)  [unwired: 1 out]
      }
      frame "Wait_for_finished" {
      }
      frame "Change_storage" {
        n172 = Variant To Data(error in=w486, type=T14 {"Autosave"=FALSE, "Path"=path "D:/"} ("Storage parameters"), Variant=w484) -> (data=w482:T14, error out=w485:errorcluster)
        n173 = Bundle By Name(cluster=w481, "Storage parameters"=w482) -> (w479:T18)
        n174 = To Variant(anything=w479) -> (Variant=w483:variant)
        n175 = Bundle(cluster=T20 {"Control_process_state_enum"=enum."Change_parameters", "variant"=variant} ("Control_process_state_cluster"), "variant"=w483) -> (w490:T20)  [unwired: 1 in]
        n176 = call "send_to_process.vi"("error in"=w485, "Control_process_state_cluster in"=w490, "Process name"="storage", "Process_communication in"=w489) -> ("error out"=w491:errorcluster, "Process_communication out"=w487:variant)  [unwired: 6 in]
      }
      frame "Change_pixelmap" {
        n177 = Variant To Data(error in=w506, type=T19 {"Mapping corrections"={"Phase increase"=0.0, "Amplitude correction"=0.0}, "Smoothing coefficients"={"Coeff 1"=0.0, "Coeff 2"=0.0}, "Fiber parameters pixelmapper"={"Frequency"=0.0, "Amplitude X"=0.0, "Amplitude Y"=0.0, "Initial Amplitude X"=0.0, "Initial Amplitude Y"=0.0, "Phase"=0.0, "Ramp type"=enum."Linear"}} ("output cluster"), Variant=w504) -> (data=w502:T19, error out=w505:errorcluster)
        n178 = Unbundle(w502) -> ("Mapping corrections"=w497:T12, "Smoothing coefficients"=w498:T11, "Fiber parameters pixelmapper"=w499:T2)
        n179 = Bundle By Name(cluster=w503, "Mapping corrections"=w497, "Smooth_coeffs_cluster"=w498, "Fiber parameters pixel_mapper"=w499) -> (w501:T18)
        n180 = To Variant(anything=w501) -> (Variant=w518:variant)
        n181 = case "Running?" shown="True" w519 {
          tunnel: w505 -> [w532 w538]
          tunnel: [w532 w537] -> w515
          tunnel: w512 -> [w531 w535]
          tunnel: [w531 w534] -> w511
          tunnel: "pixel_mapper" ("Process name") -> [w530 w533]
          tunnel: [w530 w533] -> w509
          frame False {
          }
          frame True {
            n182 = call "send_to_process.vi"("error in"=w538, "Control_process_state_cluster in"=T20 {"Control_process_state_enum"=enum."Stop", "variant"=variant} ("Control_process_state_cluster"), "Process name"=w533, "Process_communication in"=w535) -> ("error out"=w537:errorcluster, "Process_communication out"=w534:variant)  [unwired: 6 in]
          }
        }
        n183 = Bundle(cluster=T20 {"Control_process_state_enum"=enum."Change_parameters", "variant"=variant} ("Control_process_state_cluster"), "variant"=w518) -> (w514:T20)  [unwired: 1 in]
        n184 = call "send_to_process.vi"("error in"=w515, "Control_process_state_cluster in"=w514, "Process name"=w509, "Process_communication in"=w511) -> ("error out"=w513:errorcluster, "Process_communication out"=w508:variant)  [unwired: 6 in]
        n185 = case "Running?" shown="True" w519 {
          tunnel: w513 -> [w523 w529]
          tunnel: [w523 w528] -> w520
          tunnel: w509 -> [_ w526]
          tunnel: w508 -> [w522 w525]
          tunnel: [w522 w524] -> w507
          frame False {
          }
          frame True {
            n186 = call "send_to_process.vi"("error in"=w529, "Control_process_state_cluster in"=T20 {"Control_process_state_enum"=enum."Start", "variant"=variant} ("Control_process_state_cluster"), "Process name"=w526, "Process_communication in"=w525) -> ("error out"=w528:errorcluster, "Process_communication out"=w524:variant)  [unwired: 6 in]
          }
        }
      }
      frame "Change_averages" {
        n187 = Variant To Data(error in=w562, type=u8 0 ("Averages per frame"), Variant=w559) -> (data=w558:u8, error out=w560:errorcluster)
        n188 = Bundle By Name(cluster=w557, "Run parameters.Averages per frame"=w558) -> (w541:T18)
        n189 = case "Running?" shown="True" w556 {
          tunnel: w560 -> [w573 w579]
          tunnel: [w573 w578] -> w553
          tunnel: w550 -> [w572 w576]
          tunnel: "averager" ("Process name") -> [w571 w574]
          tunnel: [w572 w575] -> w548
          tunnel: [w571 w574] -> w546
          frame False {
          }
          frame True {
            n190 = call "send_to_process.vi"("error in"=w579, "Control_process_state_cluster in"=T20 {"Control_process_state_enum"=enum."Stop", "variant"=variant} ("Control_process_state_cluster"), "Process name"=w574, "Process_communication in"=w576) -> ("error out"=w578:errorcluster, "Process_communication out"=w575:variant)  [unwired: 6 in]
          }
        }
        n191 = Bundle(cluster=T20 {"Control_process_state_enum"=enum."Change_parameters", "variant"=variant} ("Control_process_state_cluster"), "variant"=w559) -> (w551:T20)  [unwired: 1 in]
        n192 = call "send_to_process.vi"("error in"=w553, "Control_process_state_cluster in"=w551, "Process name"=w546, "Process_communication in"=w548) -> ("error out"=w552:errorcluster, "Process_communication out"=w547:variant)  [unwired: 6 in]
        n193 = case "Running?" shown="True" w556 {
          tunnel: w552 -> [w564 w569]
          tunnel: [w564 w570] -> w544
          tunnel: w547 -> [w563 w567]
          tunnel: w546 -> [_ w566]
          tunnel: [w563 w565] -> w545
          frame False {
          }
          frame True {
            n194 = call "send_to_process.vi"("error in"=w569, "Control_process_state_cluster in"=T20 {"Control_process_state_enum"=enum."Start", "variant"=variant} ("Control_process_state_cluster"), "Process name"=w566, "Process_communication in"=w567) -> ("error out"=w570:errorcluster, "Process_communication out"=w565:variant)  [unwired: 6 in]
          }
        }
        n195 = call "calc_scan_infos.vi"("error in"=w544, "All scan parameters"=w541) -> ("error out"=w543:errorcluster, "Scan infos"=w540:T9)  [unwired: 8 in]
        n196 = local write "Scan infos"(w540) -> ()
      }
      frame "Save" {
        n197 = Variant To Data(error in=w598, type="" ("Comment"), Variant=w597) -> (data=w581:string, error out=w587:errorcluster)
        n198 = To Variant(anything=w581) -> (Variant=w594:variant)
        n199 = Bundle(cluster=T20 {"Control_process_state_enum"=enum."Custom", "variant"=variant} ("Control_process_state_cluster"), "variant"=w594) -> (w585:T20)  [unwired: 1 in]
        n200 = call "send_to_process.vi"("error in"=w587, "Control_process_state_cluster in"=w585, "Process name"="storage", "Process_communication in"=w583) -> ("error out"=w586:errorcluster, "Process_communication out"=w582:variant)  [unwired: 6 in]
        n201 = Unbundle By Name(w593) -> ("Save"=w591:refnum<vi>)
        n202 = property class="Bool (strict)"(reference=w591, error in=w586, "Value"=FALSE) -> (error out=w592:errorcluster)  [unwired: 1 out]
      }
      frame "Run_finished" {
        n203 = Unbundle By Name(w614) -> ("Start single"=w608:refnum<vi>, "Start cont"=w611:refnum<vi>)
        n204 = property class="Bool (strict)"(reference=w611, error in=w612, "DisabledEnum"=T24."Enabled" ("Disabled")) -> (error out=w610:errorcluster)  [unwired: 1 out]
        n205 = property class="Bool (strict)"(reference=w608, error in=w610, "Value"=FALSE) -> (error out=w609:errorcluster)  [unwired: 1 out]
        n206 = To Variant(anything=FALSE) -> (Variant=w603:variant)
        n207 = Bundle(cluster=T15 {"Main_state_enum"=enum."Shutter", "State_data_variant"=variant} ("Main_state_cluster"), "State_data_variant"=w603) -> (w604:T15)  [unwired: 1 in]
        n208 = Build Array(w604) -> (w606:T15[])
      }
      frame "Change_runmode" {
        n209 = Variant To Data(error in=w632, type=run_mode_enum."Continuous" ("Run parameters.Run mode"), Variant=w631) -> (data=w629:T6, error out=w627:errorcluster)
        n210 = Bundle By Name(cluster=w628, "Run parameters.Run mode"=w629) -> (w619:T18)
        n211 = To Variant(anything=w619) -> (Variant=w620:variant)
        n212 = Bundle(cluster=T20 {"Control_process_state_enum"=enum."Change_parameters", "variant"=variant} ("Control_process_state_cluster in"), "variant"=w620) -> (w621:T20)  [unwired: 1 in]
        n213 = call "send_to_process.vi"("error in"=w627, "Control_process_state_cluster in"=w621, "Process name"="DAQ", "Process_communication in"=w625) -> ("error out"=w626:errorcluster, "Process_communication out"=w624:variant)  [unwired: 6 in]
      }
      frame "PMT" {
        n214 = Variant To Data(error in=w651, type=TRUE, Variant=w650) -> (data=w636:bool, error out=w642:errorcluster)
        n215 = call-poly <vilib>:"DAQmx Create Virtual Channel.vi"("lines"="PMT digital line", "error in"=w642) -> ("task out"=w648:refnum<k21>, "error out"=w647:errorcluster)  [unwired: 12 in]
        n216 = call <vilib>:"DAQmx Start Task.vi"("task/channels in"=w648, "error in"=w647) -> ("task out"=w646:refnum<k21>, "error out"=w645:errorcluster)  [unwired: 12 in]
        n217 = call-poly <vilib>:"DAQmx Write.vi"("task/channels in"=w646, "data"=w636, "error in"=w645) -> ("task out"=w644:refnum<k21>, "error out"=w643:errorcluster)  [unwired: 10 in, 1 out]
        n218 = call <vilib>:"DAQmx Clear Task.vi"("task in"=w644, "error in"=w643) -> ("error out"=w639:errorcluster)  [unwired: 13 in]
        n219 = Unbundle By Name(w640) -> ("PMT"=w637:refnum<vi>)
        n220 = property class="Bool (strict)"(reference=w637, error in=w639, "Value"=w636) -> (error out=w638:errorcluster)  [unwired: 1 out]
      }
    }
    n221 = call "main_queque_manager.vi"("error in"=w205, "State insert position"=w195, "New states array"=w201, "Main state queue in"=w202) -> ("error out"=w204:errorcluster, "Main state queue out"=w203:refnum<queue>)  [unwired: 6 in]
  }
  n222 = constructor class="PerformanceCounter"(error in=w6) -> (reference out=w23:refnum<k24>, error out=w29:errorcluster)  [unwired: 2 in, 1 out]
  n223 = property class="PerformanceCounter"(reference=w23, error in=w29, "CategoryName"="Processor", "CounterName"="% Processor Time", "InstanceName"="_Total") -> (reference out=w24:refnum<k24>, error out=w25:errorcluster)
  n224 = while {
    tunnel: w24 -> [w668]
    tunnel: [w667] -> w20
    shift-right: [w665] -> w21
    shift-left: w25 -> [w669]
    shift-right: [w666] -> _
    shift-left: w22 -> [w662]
    shift-left: w22 -> [w661]
    shift-left: w22 -> [w660]
    stop <- w663 stop-if-true
    n225 = Compound Arithmetic op=ADD(w662, w661, w660) -> (w659:sgl)
    n226 = Divide(x=w659, y=sgl 3.0) -> (x/y=→"CPU":sgl)
    n227 = invoke class="PerformanceCounter" method="NextValue"(reference=w668, error in=w669) -> (reference out=w667:refnum<k24>, error out=w665:errorcluster, "NextValue"=w666:sgl)  [unwired: 1 in]
    n228 = global read "global_exit.vi" "Global_exit"() -> (w664:bool)
    n229 = Wait Until Next ms Multiple(millisecond multiple=u32 250) -> ()  [unwired: 1 out]
    n230 = Or(x=w665, y=w664) -> (x .or. y?=w663:bool)
  }
  n231 = Close Reference(reference=w20, error in (no error)=w21) -> (error out=w2:errorcluster)
  n232 = Release Queue(queue=w40, error in (no error)=w41) -> (error out=w39:errorcluster)  [unwired: 1 in, 2 out]
  n233 = Merge Errors(w38, w39, w2) -> ()  [unwired: 1 out]
  "Loaded process names" <- w10
